vi "Outlier Check.vi"(8 "error in (no error)":errorcluster, 9 "New Hours":dbl[](array[numeric]), 11 "New Data":dbl[](array[numeric])) -> (0 "error out":errorcluster, 3 "Check New Data Point 2":T1={"XY Graph 2"=[{[{0.0, "Numeric"=0.97}, {1000.0, "Numeric"=0.9733}, {2000.0, "Numeric"=0.97}, {3000.0, "Numeric"=0.97}]}, {[{4000.0, "Numeric"=0.97346}]}, {[{0.0, "Numeric"=0.9713197181503324}, {1000.0, "Numeric"=0.970989831390721}, {2000.0, "Numeric"=0.9706600566696818}, {3000.0, "Numeric"=0.9703303939491632}, {4000.0, "Numeric"=0.9700008431911267}]}, {[{0.0, "Numeric"=0.9822728418829588}, {1000.0, "Numeric"=0.9805677813713304}, {2000.0, "Numeric"=0.9802376627629179}, {3000.0, "Numeric"=0.9812824860577213}, {4000.0, "Numeric"=0.9837022512557407}]}, {[{0.0, "Numeric"=0.9603665944139}, {1000.0, "Numeric"=0.9614118814215039}, {2000.0, "Numeric"=0.9610824505649396}, {3000.0, "Numeric"=0.9593783018442069}, {4000.0, "Numeric"=0.9562994352593058}]}], "Out of Range"=FALSE})   [LabVIEW 2013, in "Data Trends.lvlib"]
uses:
  Data Trends.lvlib
  Check New Data Point.ctl
  <vilib>/Analysis/6fits.llb/Curve Fitting Criteria.ctl
  <vilib>/Analysis/NI_AALPro.lvlib
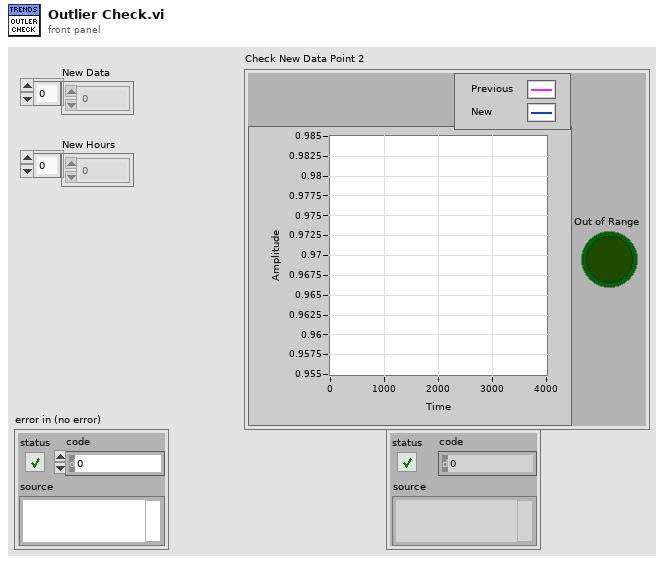
[diagram p1: front panel]
types:
  T1 = typedef "Data Trends.lvlib/Check New Data Point.ctl" = cluster{"XY Graph 2":cluster{cluster{dbl, "Numeric":dbl}[]}[], "Out of Range":bool}
  T2 = typedef "NI_AALPro.lvlib/Curve Fitting Criteria.ctl" = u16
  T3 = cluster{"Lower Bound (out)":cluster{dbl, "p(x)":dbl}[]}[]
  T4 = cluster{cluster{"Lower Bound (out)":cluster{dbl, "p(x)":dbl}[]}[], "Out of Range?":bool}
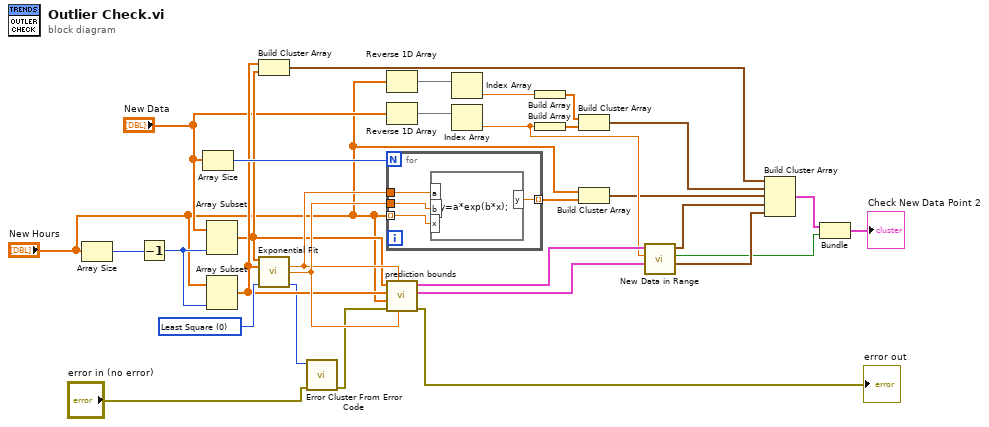
[diagram p0: block diagram]
diagram:
  w26 = T2 0 items=["Least Square", "Least Absolute Residual", "Bisquare"] ("method")
  n1 = Array Size(array="New Hours") -> (size(s)=w27:i32)
  n2 = Decrement(x=w27) -> (x-1=w28:i32)
  n3 = Array Size(array="New Data") -> (size(s)=w29:i32)
  n4 = Array Subset(array="New Data", length=w28) -> (w24:dbl[])  [unwired: 1 in]
  n5 = Array Subset(array="New Hours", length=w28) -> (w25:dbl[])  [unwired: 1 in]
  n6 = Build Cluster Array(w25, w24) -> (w17:cluster{dbl, dbl}[])
  n7 = call <vilib>:"Exponential Fit.vi"("Y"=w24, "X"=w25, "method"=w26) -> ("amplitude"=w30:dbl, "damping"=w31:dbl, "error"=w15:i32)  [unwired: 7 in, 3 out]
  n8 = call <vilib>:"Error Cluster From Error Code.vi"("error in (no error)"="error in (no error)", "error code (0)"=w15) -> ("error out"=w14:errorcluster)  [unwired: 7 in]
  n9 = Reverse 1D Array(array="New Hours") -> (reversed array=w20:dbl[])
  n10 = Reverse 1D Array(array="New Data") -> (reversed array=w22:dbl[])
  n11 = for {
    N: w29 -> [_]
    tunnel: w30 -> [w35]
    tunnel: w31 -> [w34]
    tunnel: "New Hours" -> [w33] mode=indexing
    tunnel: [w32] -> w23 mode=indexing
    n12 = formula code="y=a*exp(b*x);"("a"=w35, "b"=w34, "x"=w33) -> ("y"=w32:dbl)
  }
  n13 = call "prediction bounds.vi"("damping"=w31, "amplitude"=w30, "error in (no error)"=w14, "Hours array"="New Hours", "Previous Hours Array"=w25, "Previous Data Array"=w24) -> ("error out"=→"error out":errorcluster, "Lower Bound"=w10:cluster{"Hours array":dbl[], "P(A)":dbl[]}, "Upper Bound"=w11:cluster{"Hours array":dbl[], "P(A)":dbl[]})  [unwired: 3 in]
  n14 = Index Array(array=w20) -> (element=w18:dbl)  [unwired: 1 in]
  n15 = Index Array(array=w22) -> (element=w8:dbl)  [unwired: 1 in]
  n16 = Build Array(w18) -> (w16:dbl[])
  n17 = Build Array(w8) -> (w9:dbl[])
  n18 = Build Cluster Array(w16, w9) -> (w7:cluster{dbl, dbl}[])
  n19 = Build Cluster Array("New Hours", w23) -> (w6:cluster{dbl, "y":dbl}[])
  n20 = call "New Data in Range.vi"("Lower Bound"=w10, "New Data Point"=w8, "Upper Bound"=w11) -> ("Lower Bound (out)"=w4:cluster{dbl, "p(x)":dbl}[], "Out of Range?"=w1:bool, "Upper Bound (out)"=w5:cluster{dbl, "p(x)":dbl}[])  [unwired: 6 in]
  n21 = Build Cluster Array(w17, w7, w6, w5, w4) -> (w3:T3)
  n22 = Bundle(w3, "Out of Range?"=w1) -> (→"Check New Data Point 2":T4)  [unwired: 1 in]
